vi "Assert Dynamic Methods.vi"() -> ()   [LabVIEW 2015, in "Admin_Actor.lvlib" / "Admin_Actor.lvclass"]
uses:
  Admin_Actor.lvclass
  Member_Actor/MemberPanel/MemberPanel.lvclass
  User_Actor/Member_Actor Messages/SwitchOption Msg/SwitchOption Msg.lvclass
  User_Actor/Member_Actor Messages/SwitchOption Msg/SwitchOption Msg.lvclass/SwitchOption Msg.ctl
panel:
  in  "Admin_Actor in 2":refnum<class "Admin_Actor.lvclass">
  in  "SubPanelRef":refnum<vi>
  in  "Panel Controller":refnum<class "MemberPanel.lvclass">
  in  "error in (no error)":errorcluster
  in  "Base Path":path
  in  "ThreadName(\"\")":string
  in  "Admin_Actor in":refnum<class "Admin_Actor.lvclass">
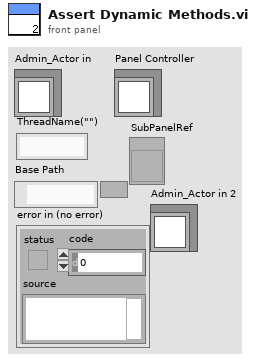
[diagram p1: front panel]
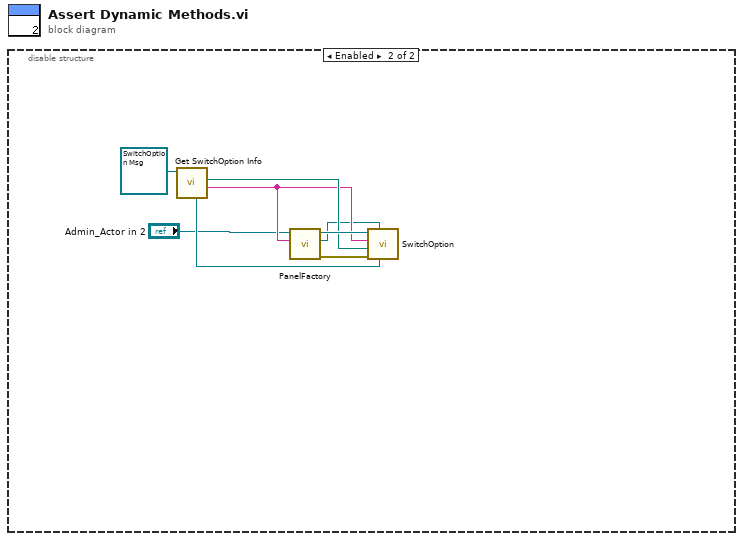
[diagram p0: block diagram]
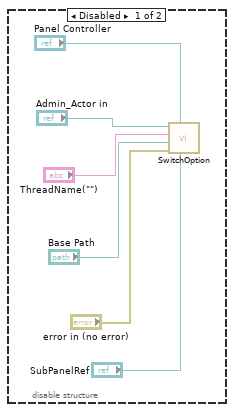
[diagram p2: hidden frame]
diagram:
  n1 = disable-structure shown="Enabled" {
    frame Disabled {
      n2 = call-dynamic "SwitchOption.vi"("SubPanelRef"="SubPanelRef", "Panel Controller"="Panel Controller", "error in (no error)"="error in (no error)", "Base Path"="Base Path", "ThreadName(\"\")"="ThreadName(\"\")", "Admin_Actor in"="Admin_Actor in") -> ()  [unwired: 4 in, 2 out]
    }
    frame Enabled {
      n3 = call "Get SwitchOption Info.vi"("SwitchOption Msg in"=refnum<class "SwitchOption Msg.lvclass"> refnum) -> ("ThreadName(\"\")"=w10:string, "Base Path"=w12:path, "SubPanelRef"=w11:refnum<vi>)  [unwired: 6 in, 2 out]
      n4 = call-dynamic "PanelFactory.vi"("ThreadName(\"\")"=w10, "Admin_Actor in"="Admin_Actor in 2") -> ("error out"=w14:errorcluster, "MemberPanel(Product)"=w9:refnum<class "MemberPanel.lvclass">, "Admin_Actor out"=w13:refnum<class "Admin_Actor.lvclass">)  [unwired: 7 in]
      n5 = call-dynamic "SwitchOption.vi"("SubPanelRef"=w11, "Panel Controller"=w9, "error in (no error)"=w14, "Base Path"=w12, "ThreadName(\"\")"=w10, "Admin_Actor in"=w13) -> ()  [unwired: 4 in, 2 out]
    }
  }
